vi "Add Clocked Bit.vi"(6 "Transition action":T1=enum."<Use session default>", 8 "error in (no error)":errorcluster, 9 "Bit type":T2=enum."Data", 10 "Bit value":u8(ring)=4 items=["0", "1", "Z", "L", "H", "X", "T", "V"], 11 "I2C waveform info":T3) -> (0 "error out":errorcluster, 3 "I2C waveform info out":T3)   [LabVIEW 2009, in "IDW.lvlib"]
doc: "Adds a single bit to the I2C waveform. This is a low-level VI.\n\nFor a compare bit (<b>L</b> or <b>H</b>), the SDA line is released and a single sample in the center of the clock pulse is compared against the expected value. For a drive bit (<b>1/Z</b>, or <b>0</b>), the value is written to the SDA line according to the timing parameters specified by the <b>Init</b> VI. All other bits (X, T, V) are invalid.\n\nFor a compare bit, the <b>Bit type</b> is added to a list of compare bits along with the location of the compare sample in the waveform. These lists are output by the <b>Close</b> VI.\n\nTiming parameters that affect this waveform segment's length are: <b>tSU;DAT</b>, <b>tHIGH</b>, <b>tHD;DAT</b>, and <b>fSCL</b>."
uses:
  IDW.lvlib
  _Typedefs/Waveform info.ctl
  _Typedefs/Timing - ticks.ctl
  _Typedefs/Default transition action.ctl
  _Typedefs/Bit type.ctl
  _Typedefs/Transition action.ctl
  _Private/Polymorphics/Change Bit Value - Single.vi
  _Typedefs/Channel Ring.ctl
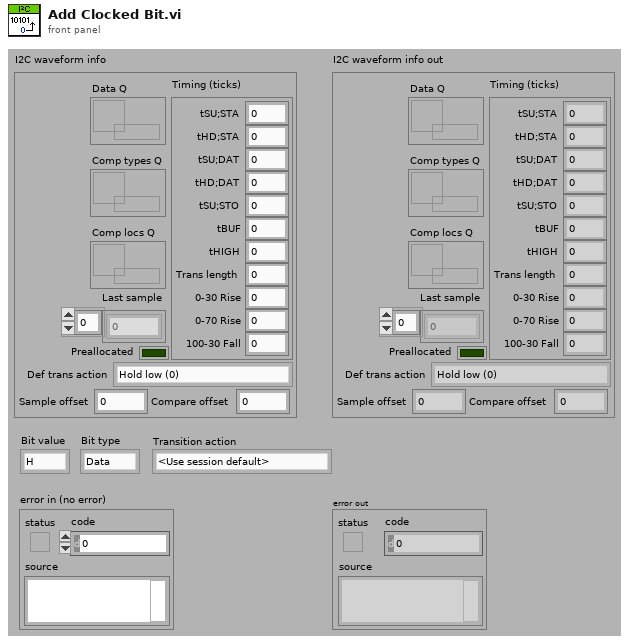
[diagram p1: front panel]
types:
  T1 = typedef "IDW.lvlib/Transition action.ctl" = enum16{"Hold low (0)", "Release (Z)", "Set up next value", "Hold previous value", "Preserve tHD;DAT and tSU;DAT", "<Use session default>"}
  T2 = typedef "IDW.lvlib/Bit type.ctl" = enum16{"ACK", "Data"}
  T3 = typedef "IDW.lvlib/Waveform info.ctl" = cluster{"Last sample":u8[], "Sample offset":u64, "Compare offset":u64, "Timing (ticks)":T4, "Preallocated":bool, "Def trans action":T5, "Data Q":refnum<queue>, "Comp types Q":refnum<queue>, "Comp locs Q":refnum<queue>}
  T4 = typedef "IDW.lvlib/Timing - ticks.ctl" = cluster{"tSU;STA":i32, "tHD;STA":i32, "tSU;DAT":i32, "tHD;DAT":i32, "tSU;STO":i32, "tBUF":i32, "tHIGH":i32, "Trans length":i32, "0-30 Rise":i32, "0-70 Rise":i32, "100-30 Fall":i32}
  T5 = typedef "IDW.lvlib/Default transition action.ctl" = enum16{"Hold low (0)", "Release (Z)", "Set up next value", "Hold previous value", "Preserve tHD;DAT and tSU;DAT"}
  T6 = typedef "IDW.lvlib/Channel Ring.ctl" = u16
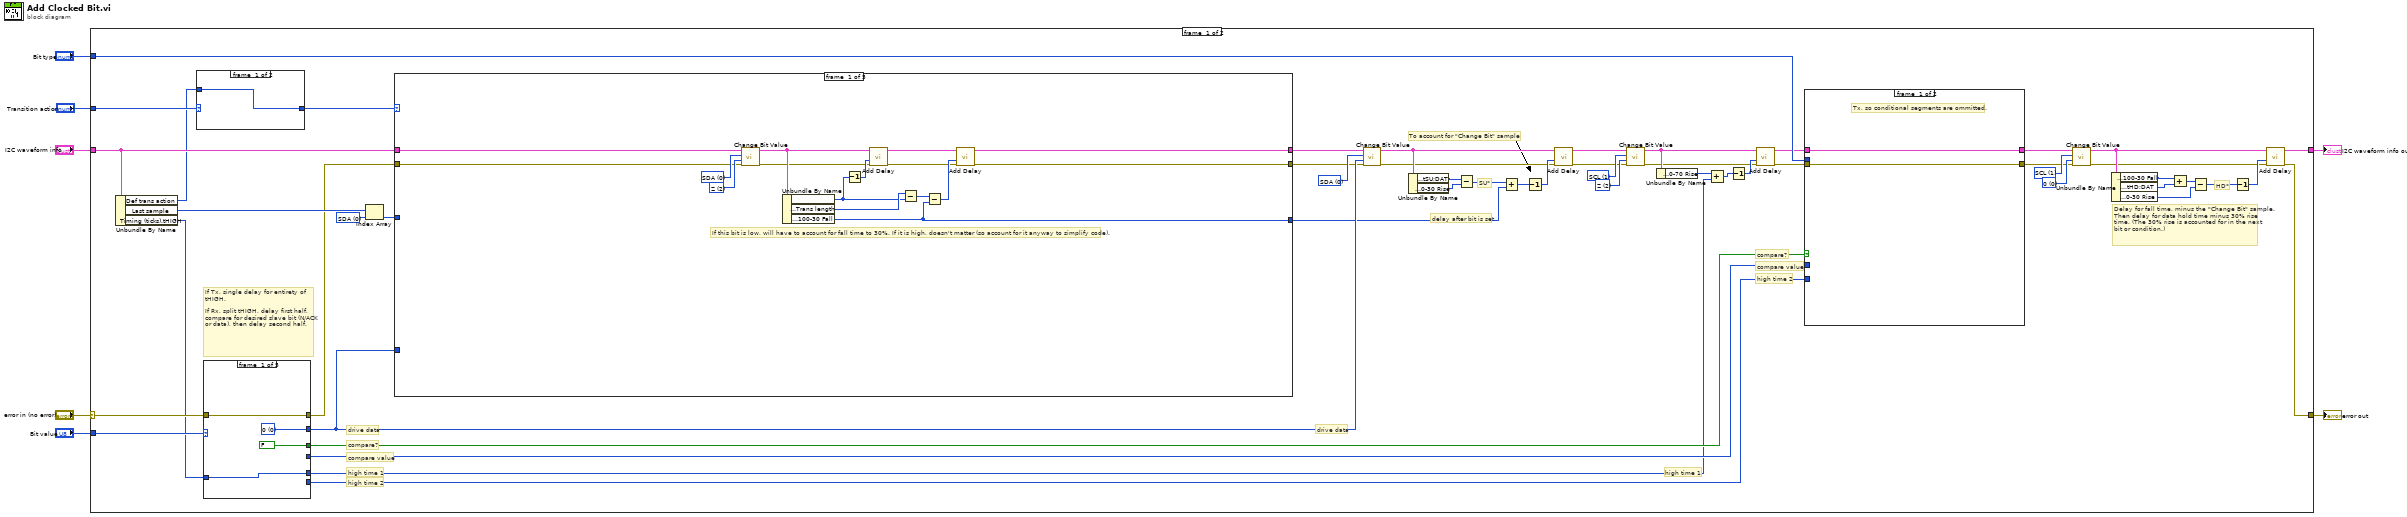
[diagram p0: block diagram]
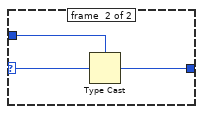
[diagram p2: hidden frame]
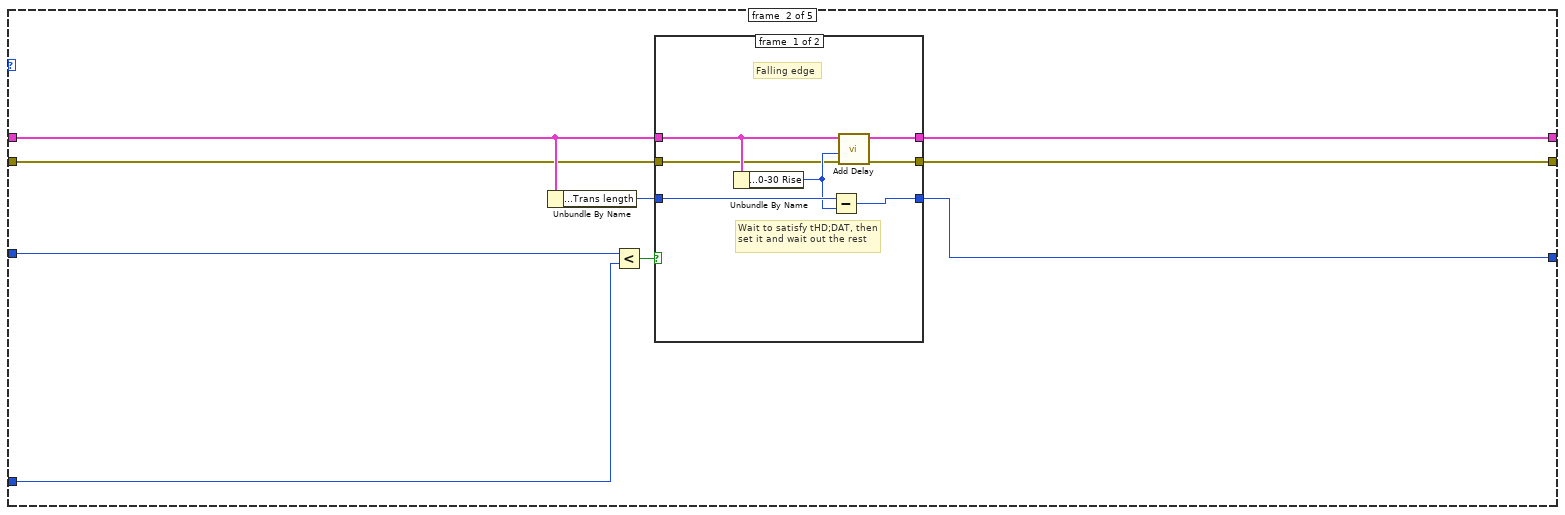
[diagram p3: hidden frame]
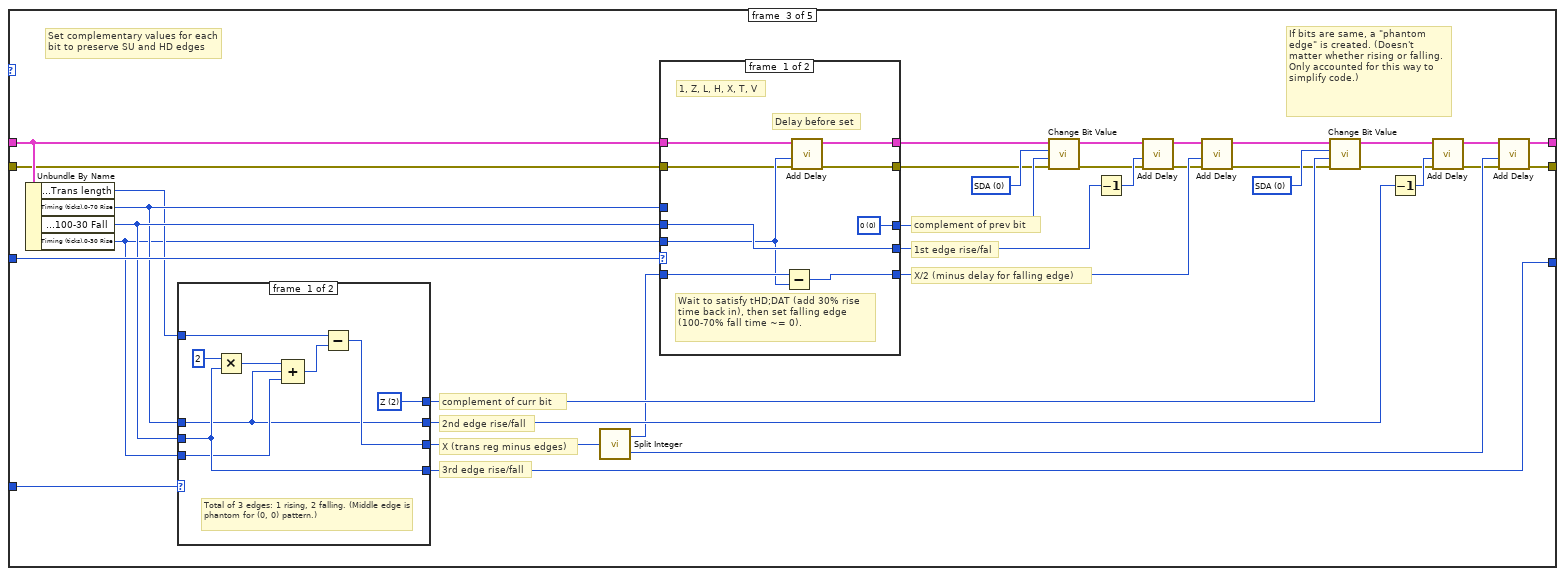
[diagram p5: hidden frame]
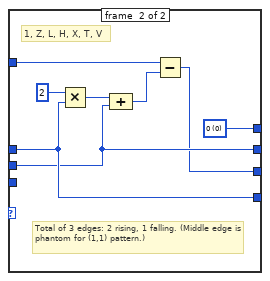
[diagram p6: hidden frame]
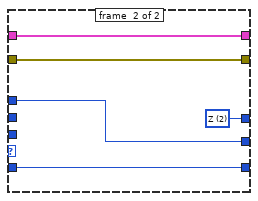
[diagram p7: hidden frame]
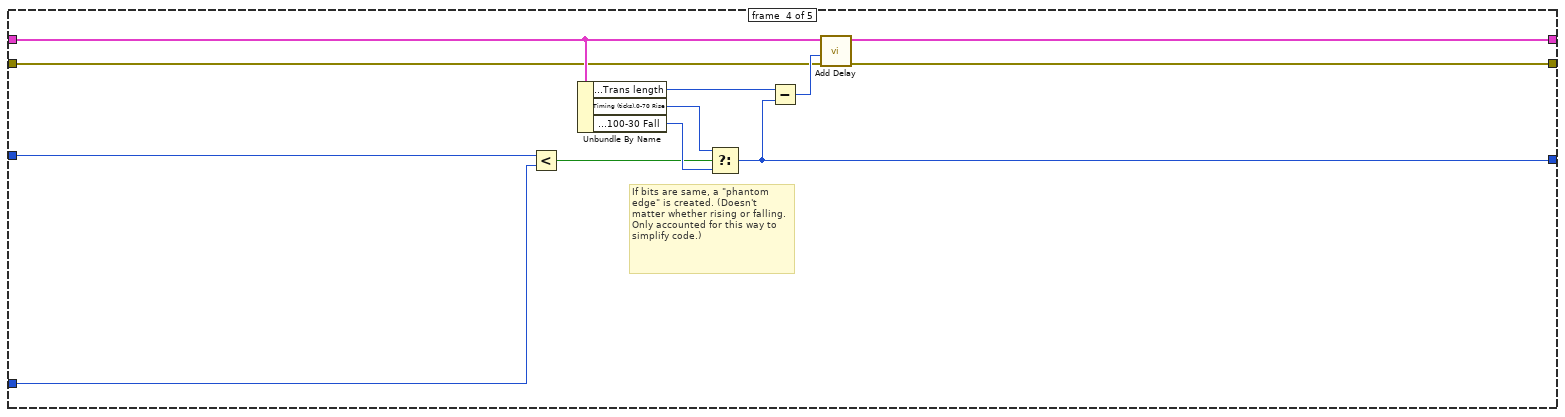
[diagram p8: hidden frame]
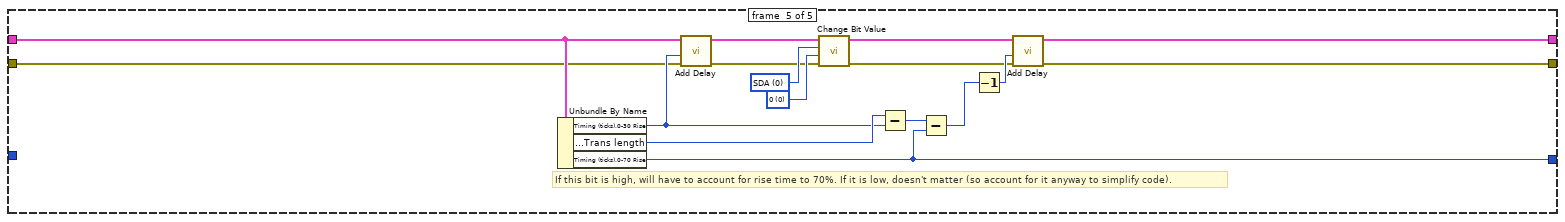
[diagram p9: hidden frame]
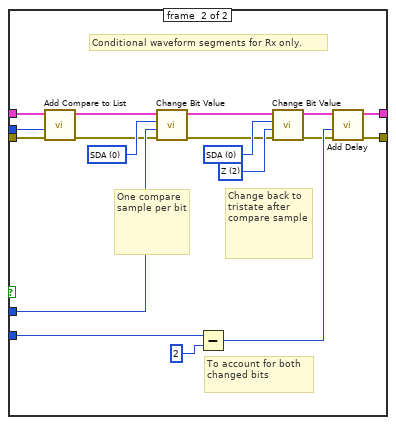
[diagram p10: hidden frame]
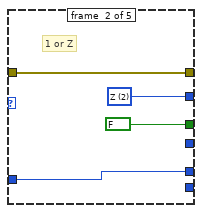
[diagram p11: hidden frame]
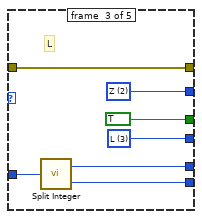
[diagram p12: hidden frame]
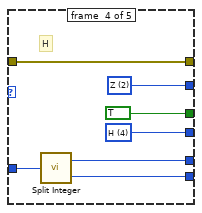
[diagram p13: hidden frame]
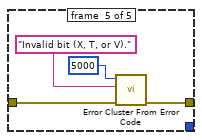
[diagram p14: hidden frame]
diagram:
  n1 = case shown="No Error" "error in (no error)" {
    selector: "error in (no error)" -> [w51 w241]
    tunnel: [w40 w240] -> w7
    tunnel: "I2C waveform info" -> [w21 w240]
    tunnel: [w8 w241] -> w4
    tunnel: "Bit value" -> [w29 _]
    tunnel: "Bit type" -> [w48 _]
    tunnel: "Transition action" -> [w20 _]
    frame #0 {
      w33 = T6 0 items=["SDA", "SCL"] ("I2C Ring")
      w38 = T6 0 items=["SDA", "SCL"] ("I2C Ring")
      w56 = u8 0 items=["0", "1", "Z", "L", "H", "X", "T", "V"] ("State")
      w57 = T6 1 items=["SDA", "SCL"] ("I2C Ring")
      w60 = u8 2 items=["0", "1", "Z", "L", "H", "X", "T", "V"] ("State")
      w59 = T6 1 items=["SDA", "SCL"] ("I2C Ring")
      # "HD*"
      # "SU*"
      # "If Tx, single delay for entirety of tHIGH.\n\nIf Rx, split tHIGH, delay first half, compare for desired slave bit (N/ACK or data), then delay second half."
      # "high time 1"
      # "drive data"
      # "high time 2"
      # "compare value"
      # "compare?"
      # "delay after bit is set"
      # "drive data"
      # "Delay for fall time, minus the \"Change Bit\" sample. Then delay for data hold time minus 30% rise time. (The 30% rise is accounted for in the next bit or condition.)"
      # "To account for \"Change Bit\" sample"
      # "high time 2"
      # "high time 1"
      # "compare value"
      # "compare?"
      n2 = Unbundle By Name(w21) -> ("Def trans action"=w17:T5, "Last sample"=w39:u8[], "Timing (ticks).tHIGH"=w18:i32)
      n3 = case shown="\"<Use session default>\"" w20 {
        selector: w20 -> [_ w64]
        tunnel: [w61 w63] -> w19
        tunnel: w17 -> [w61 w62]
        frame #0 {
        }
        frame #1 {
          n4 = Type Cast(type=w62, x=w64) -> (*(type *) &x=w63:T5)
        }
      }
      n5 = case shown="Default" w29 {
        tunnel: [w216 w220 w226 w232 _] -> w43
        tunnel: [FALSE FALSE TRUE TRUE _] -> w55
        tunnel: [_ _ w225 w234 _] -> w54
        tunnel: [_ _ w223 w230 _] -> w28
        tunnel: w18 -> [w216 w220 w227 w233 _]
        tunnel: [w215 w219 w224 w231 w238] -> w15
        tunnel: w51 -> [w215 w219 w224 w231 w239]
        tunnel: [w214 w218 w222 w229 _] -> w27
        frame #0 {
          w214 = u8 0 items=["0", "1", "Z", "L", "H", "X", "T", "V"] ("Complement")
        }
        frame #1 {
          w218 = u8 2 items=["0", "1", "Z", "L", "H", "X", "T", "V"] ("Complement")
          # "1 or Z"
        }
        frame #2 {
          w222 = u8 2 items=["0", "1", "Z", "L", "H", "X", "T", "V"] ("Complement")
          w225 = u8 3 items=["0", "1", "Z", "L", "H", "X", "T", "V"] ("Bit")
          # "L"
          n6 = call "Split Integer.vi"("Input"=w227) -> ("First half"=w226:i32, "Second half"=w223:i32)
        }
        frame #3 {
          w229 = u8 2 items=["0", "1", "Z", "L", "H", "X", "T", "V"] ("Complement")
          w234 = u8 4 items=["0", "1", "Z", "L", "H", "X", "T", "V"] ("Bit")
          # "H"
          n7 = call "Split Integer.vi"("Input"=w233) -> ("First half"=w232:i32, "Second half"=w230:i32)
        }
        frame #4 {
          n8 = call <vilib>:"Error Cluster From Error Code.vi"("error in (no error)"=w239, "error message (\"\")"="Invalid bit (X, T, or V)." ("error message (\"\")"), "error code (0)"=5000) -> ("error out"=w238:errorcluster)  [unwired: 1 in, 5 out]
        }
      }
      n9 = Index Array(array=w39, index=w38) -> (element=w37:u8)
      n10 = case shown="\"Hold previous value\"" w19 {
        tunnel: [w69 w84 w110 w169 w183] -> w32
        tunnel: w21 -> [w77 w89 w118 w176 w186]
        tunnel: w37 -> [_ w87 w130 w172 _]
        tunnel: [w70 w85 w109 w170 w182] -> w23
        tunnel: w27 -> [_ w83 w108 w168 _]
        tunnel: [w66 w82 w101 w167 w179] -> w16
        tunnel: w15 -> [w65 w81 w100 w166 w178]
        frame #0 {
          w79 = u8 2 items=["0", "1", "Z", "L", "H", "X", "T", "V"] ("State")
          w80 = T6 0 items=["SDA", "SCL"] ("I2C Ring")
          # "If this bit is low, will have to account for fall time to 30%. If it is high, doesn't matter (so account for it anyway to simplify code)."
          n11 = call-poly "Change Bit Value.vi"("error in (no error)"=w65, "State"=w79, "Bit"=w80, "I2C waveform info"=w77) -> ("error out"=w68:errorcluster, "I2C waveform info out"=w74:T3)  [unwired: 6 out]
          n12 = Unbundle By Name(w74) -> ("Timing (ticks).0-70 Rise"=w72:i32, "Timing (ticks).Trans length"=w75:i32, "Timing (ticks).100-30 Fall"=w70:i32)
          n13 = Decrement(x=w72) -> (x-1=w73:i32)
          n14 = call "Add Delay.vi"("error in (no error)"=w68, "# Samples"=w73, "I2C waveform info"=w74) -> ("error out"=w67:errorcluster, "I2C waveform info out"=w76:T3)  [unwired: 1 in, 6 out]
          n15 = Subtract(x=w75, y=w72) -> (x-y=w78:i32)
          n16 = Subtract(x=w78, y=w70) -> (x-y=w71:i32)
          n17 = call "Add Delay.vi"("error in (no error)"=w67, "# Samples"=w71, "I2C waveform info"=w76) -> ("error out"=w66:errorcluster, "I2C waveform info out"=w69:T3)  [unwired: 1 in, 6 out]
        }
        frame #1 {
          n18 = Unbundle By Name(w89) -> ("Timing (ticks).Trans length"=w88:i32)
          n19 = Less?(x=w87, y=w83) -> (x < y?=w86:bool)
          n20 = case shown="False" w86 {
            tunnel: w89 -> [w93 w99]
            tunnel: [w95 w99] -> w84
            tunnel: [w96 w98] -> w85
            tunnel: w88 -> [w94 w98]
            tunnel: [w91 w97] -> w82
            tunnel: w81 -> [w90 w97]
            frame #0 {
              # "Falling edge"
              # "Wait to satisfy tHD;DAT, then set it and wait out the rest"
              n21 = Unbundle By Name(w93) -> ("Timing (ticks).0-30 Rise"=w92:i32)
              n22 = Subtract(x=w94, y=w92) -> (x-y=w96:i32)
              n23 = call "Add Delay.vi"("error in (no error)"=w90, "# Samples"=w92, "I2C waveform info"=w93) -> ("error out"=w91:errorcluster, "I2C waveform info out"=w95:T3)  [unwired: 1 in, 6 out]
            }
            frame #1 {
              # "Rising edge, or \"phantom edge\" for (0,0) and (1,1). Doesn't matter whether phantom is rising or falling. Only accounted for this way to simplify code."
            }
          }
        }
        frame #2 {
          w128 = T6 0 items=["SDA", "SCL"] ("I2C Ring")
          w133 = T6 0 items=["SDA", "SCL"] ("I2C Ring")
          # "X/2 (minus delay for falling edge)"
          # "1st edge rise/fal"
          # "complement of prev bit"
          # "complement of curr bit"
          # "3rd edge rise/fall"
          # "X (trans reg minus edges)"
          # "2nd edge rise/fall"
          # "If bits are same, a \"phantom edge\" is created. (Doesn't matter whether rising or falling. Only accounted for this way to simplify code.)"
          # "Set complementary values for each bit to preserve SU and HD edges"
          n24 = Unbundle By Name(w118) -> ("Timing (ticks).Trans length"=w115:i32, "Timing (ticks).0-70 Rise"=w116:i32, "Timing (ticks).100-30 Fall"=w117:i32, "Timing (ticks).0-30 Rise"=w114:i32)
          n25 = case shown="1.." w108 {
            tunnel: [w143 w151] -> w127
            tunnel: [w135 w146] -> w121
            tunnel: [w137 w144] -> w113
            tunnel: [w142 w147] -> w109
            tunnel: w115 -> [w138 w150]
            tunnel: w117 -> [w142 w146]
            tunnel: w116 -> [w135 w147]
            tunnel: w114 -> [w140 _]
            frame #0 {
              w143 = u8 2 items=["0", "1", "Z", "L", "H", "X", "T", "V"] ("Complement")
              # "Total of 3 edges: 1 rising, 2 falling. (Middle edge is phantom for (0, 0) pattern.)"
              n26 = Multiply(x=2, y=w142) -> (x*y=w136:i32)
              n27 = Compound Arithmetic op=ADD(w136, w135, w140) -> (w139:i32)
              n28 = Subtract(x=w138, y=w139) -> (x-y=w137:i32)
            }
            frame #1 {
              w151 = u8 0 items=["0", "1", "Z", "L", "H", "X", "T", "V"] ("Complement")
              # "1, Z, L, H, X, T, V"
              # "Total of 3 edges: 2 rising, 1 falling. (Middle edge is phantom for (1,1) pattern.)"
              n29 = Multiply(x=2, y=w147) -> (x*y=w148:i32)
              n30 = Compound Arithmetic op=ADD(w148, w146) -> (w145:i32)
              n31 = Subtract(x=w150, y=w145) -> (x-y=w144:i32)
            }
          }
          n32 = call "Split Integer.vi"("Input"=w113) -> ("First half"=w112:i32, "Second half"=w111:i32)
          n33 = case shown="1.." w130 {
            tunnel: w118 -> [w156 w165]
            tunnel: [w159 w165] -> w132
            tunnel: [w160 w163] -> w119
            tunnel: [w158 w164] -> w129
            tunnel: w112 -> [w157 w163]
            tunnel: [w155 w162] -> w122
            tunnel: w116 -> [_ w162]
            tunnel: w117 -> [w155 _]
            tunnel: w114 -> [w154 _]
            tunnel: [w153 w161] -> w102
            tunnel: w100 -> [w152 w161]
            frame #0 {
              w158 = u8 0 items=["0", "1", "Z", "L", "H", "X", "T", "V"] ("Complement")
              # "1, Z, L, H, X, T, V"
              # "Delay before set"
              # "Wait to satisfy tHD;DAT (add 30% rise time back in), then set falling edge (100-70% fall time ~= 0)."
              n34 = Subtract(x=w157, y=w154) -> (x-y=w160:i32)
              n35 = call "Add Delay.vi"("error in (no error)"=w152, "# Samples"=w154, "I2C waveform info"=w156) -> ("error out"=w153:errorcluster, "I2C waveform info out"=w159:T3)  [unwired: 1 in, 6 out]
            }
            frame #1 {
              w164 = u8 2 items=["0", "1", "Z", "L", "H", "X", "T", "V"] ("Complement")
            }
          }
          n36 = call-poly "Change Bit Value.vi"("error in (no error)"=w102, "State"=w129, "Bit"=w133, "I2C waveform info"=w132) -> ("error out"=w103:errorcluster, "I2C waveform info out"=w131:T3)  [unwired: 6 out]
          n37 = Decrement(x=w122) -> (x-1=w134:i32)
          n38 = call "Add Delay.vi"("error in (no error)"=w103, "# Samples"=w134, "I2C waveform info"=w131) -> ("error out"=w107:errorcluster, "I2C waveform info out"=w124:T3)  [unwired: 1 in, 6 out]
          n39 = call "Add Delay.vi"("error in (no error)"=w107, "# Samples"=w119, "I2C waveform info"=w124) -> ("error out"=w106:errorcluster, "I2C waveform info out"=w123:T3)  [unwired: 1 in, 6 out]
          n40 = call-poly "Change Bit Value.vi"("error in (no error)"=w106, "State"=w127, "Bit"=w128, "I2C waveform info"=w123) -> ("error out"=w105:errorcluster, "I2C waveform info out"=w125:T3)  [unwired: 6 out]
          n41 = Decrement(x=w121) -> (x-1=w126:i32)
          n42 = call "Add Delay.vi"("error in (no error)"=w105, "# Samples"=w126, "I2C waveform info"=w125) -> ("error out"=w104:errorcluster, "I2C waveform info out"=w120:T3)  [unwired: 1 in, 6 out]
          n43 = call "Add Delay.vi"("error in (no error)"=w104, "# Samples"=w111, "I2C waveform info"=w120) -> ("error out"=w101:errorcluster, "I2C waveform info out"=w110:T3)  [unwired: 1 in, 6 out]
        }
        frame #3 {
          # "If bits are same, a \"phantom edge\" is created. (Doesn't matter whether rising or falling. Only accounted for this way to simplify code.)"
          n44 = Less?(x=w172, y=w168) -> (x < y?=w171:bool)
          n45 = Unbundle By Name(w176) -> ("Timing (ticks).Trans length"=w175:i32, "Timing (ticks).0-70 Rise"=w174:i32, "Timing (ticks).100-30 Fall"=w173:i32)
          n46 = Select(t=w174, s=w171, f=w173) -> (s? t:f=w170:i32)
          n47 = Subtract(x=w175, y=w170) -> (x-y=w177:i32)
          n48 = call "Add Delay.vi"("error in (no error)"=w166, "# Samples"=w177, "I2C waveform info"=w176) -> ("error out"=w167:errorcluster, "I2C waveform info out"=w169:T3)  [unwired: 1 in, 6 out]
        }
        frame #4 {
          w191 = u8 0 items=["0", "1", "Z", "L", "H", "X", "T", "V"] ("State")
          w192 = T6 0 items=["SDA", "SCL"] ("I2C Ring")
          # "If this bit is high, will have to account for rise time to 70%. If it is low, doesn't matter (so account for it anyway to simplify code)."
          n49 = Unbundle By Name(w186) -> ("Timing (ticks).0-30 Rise"=w184:i32, "Timing (ticks).Trans length"=w185:i32, "Timing (ticks).0-70 Rise"=w182:i32)
          n50 = call "Add Delay.vi"("error in (no error)"=w178, "# Samples"=w184, "I2C waveform info"=w186) -> ("error out"=w181:errorcluster, "I2C waveform info out"=w189:T3)  [unwired: 1 in, 6 out]
          n51 = call-poly "Change Bit Value.vi"("error in (no error)"=w181, "State"=w191, "Bit"=w192, "I2C waveform info"=w189) -> ("error out"=w180:errorcluster, "I2C waveform info out"=w193:T3)  [unwired: 6 out]
          n52 = Subtract(x=w185, y=w184) -> (x-y=w188:i32)
          n53 = Subtract(x=w188, y=w182) -> (x-y=w187:i32)
          n54 = Decrement(x=w187) -> (x-1=w190:i32)
          n55 = call "Add Delay.vi"("error in (no error)"=w180, "# Samples"=w190, "I2C waveform info"=w193) -> ("error out"=w179:errorcluster, "I2C waveform info out"=w183:T3)  [unwired: 1 in, 6 out]
        }
      }
      n56 = call-poly "Change Bit Value.vi"("error in (no error)"=w16, "State"=w27, "Bit"=w33, "I2C waveform info"=w32) -> ("error out"=w14:errorcluster, "I2C waveform info out"=w31:T3)  [unwired: 6 out]
      n57 = Unbundle By Name(w31) -> ("Timing (ticks).tSU;DAT"=w26:i32, "Timing (ticks).0-30 Rise"=w25:i32)
      n58 = Subtract(x=w26, y=w25) -> (x-y=w24:i32)
      n59 = Add(x=w24, y=w23) -> (x+y=w22:i32)
      n60 = Decrement(x=w22) -> (x-1=w30:i32)
      n61 = call "Add Delay.vi"("error in (no error)"=w14, "# Samples"=w30, "I2C waveform info"=w31) -> ("error out"=w13:errorcluster, "I2C waveform info out"=w58:T3)  [unwired: 1 in, 6 out]
      n62 = call-poly "Change Bit Value.vi"("error in (no error)"=w13, "State"=w60, "Bit"=w59, "I2C waveform info"=w58) -> ("error out"=w12:errorcluster, "I2C waveform info out"=w47:T3)  [unwired: 6 out]
      n63 = Unbundle By Name(w47) -> ("Timing (ticks).0-70 Rise"=w44:i32)
      n64 = Add(x=w44, y=w43) -> (x+y=w41:i32)
      n65 = Decrement(x=w41) -> (x-1=w50:i32)
      n66 = call "Add Delay.vi"("error in (no error)"=w12, "# Samples"=w50, "I2C waveform info"=w47) -> ("error out"=w11:errorcluster, "I2C waveform info out"=w42:T3)  [unwired: 1 in, 6 out]
      n67 = case shown="True" w55 {
        tunnel: [w195 w211] -> w53
        tunnel: w42 -> [w195 w204]
        tunnel: w54 -> [_ w212]
        tunnel: w28 -> [_ w206]
        tunnel: w48 -> [_ w201]
        tunnel: w11 -> [w194 w200]
        tunnel: [w194 w196] -> w10
        frame #0 {
          # "Tx, so conditional segments are ommitted."
        }
        frame #1 {
          w208 = u8 2 items=["0", "1", "Z", "L", "H", "X", "T", "V"] ("State")
          w210 = T6 0 items=["SDA", "SCL"] ("I2C Ring")
          w213 = T6 0 items=["SDA", "SCL"] ("I2C Ring")
          # "To account for both changed bits"
          # "Change back to tristate after compare sample"
          # "One compare sample per bit"
          # "Conditional waveform segments for Rx only."
          n68 = call "Add Compare to List.vi"("error in (no error)"=w200, "Bit type"=w201, "I2C waveform info"=w204) -> ("error out"=w199:errorcluster, "I2C waveform info out"=w203:T3)  [unwired: 7 out]
          n69 = call-poly "Change Bit Value.vi"("error in (no error)"=w199, "State"=w212, "Bit"=w213, "I2C waveform info"=w203) -> ("error out"=w198:errorcluster, "I2C waveform info out"=w202:T3)  [unwired: 6 out]
          n70 = Subtract(x=w206, y=2) -> (x-y=w205:i32)
          n71 = call-poly "Change Bit Value.vi"("error in (no error)"=w198, "State"=w208, "Bit"=w210, "I2C waveform info"=w202) -> ("error out"=w197:errorcluster, "I2C waveform info out"=w209:T3)  [unwired: 6 out]
          n72 = call "Add Delay.vi"("error in (no error)"=w197, "# Samples"=w205, "I2C waveform info"=w209) -> ("error out"=w196:errorcluster, "I2C waveform info out"=w211:T3)  [unwired: 1 in, 6 out]
        }
      }
      n73 = call-poly "Change Bit Value.vi"("error in (no error)"=w10, "State"=w56, "Bit"=w57, "I2C waveform info"=w53) -> ("error out"=w9:errorcluster, "I2C waveform info out"=w52:T3)  [unwired: 6 out]
      n74 = Unbundle By Name(w52) -> ("Timing (ticks).100-30 Fall"=w46:i32, "Timing (ticks).tHD;DAT"=w45:i32, "Timing (ticks).0-30 Rise"=w35:i32)
      n75 = Add(x=w46, y=w45) -> (x+y=w36:i32)
      n76 = Subtract(x=w36, y=w35) -> (x-y=w34:i32)
      n77 = Decrement(x=w34) -> (x-1=w49:i32)
      n78 = call "Add Delay.vi"("error in (no error)"=w9, "# Samples"=w49, "I2C waveform info"=w52) -> ("error out"=w8:errorcluster, "I2C waveform info out"=w40:T3)  [unwired: 1 in, 6 out]
    }
    frame #1 {
      (unwired) u64 0 ("Offset")
    }
  }
  "I2C waveform info out" <- w7
  "error out" <- w4
